vi "Send Open Front Panel.vi"(5 "Activate?":bool, 7 "Priority":T2=enum."Normal" caption="Message Priority (Normal)", 8 "error in (no error)":errorcluster, 9 "Front Panel Window:State":T1(ring), 10 "View Hierarchy Level":i32, 11 "Message Enqueuer in":refnum<class "Message Enqueuer.lvclass">) -> (0 "error out":errorcluster, 3 "Message Enqueuer out":refnum<class "Message Enqueuer.lvclass">)   [LabVIEW 2023, in "GUI Views.lvlib" / "Open Front Panel Msg.lvclass"]
doc: "Sends the <b>GUI Views.lvlib:Open Front Panel Msg.lvclass</b> message.\n\nThis message will call <b>Open Front Panel.vi</b> on the <b>GUI Views.lvlib:GUI View.lvclass</b> actor.\n\n<b>Open Front Panel.vi Description</b>\nOpens the Front Panel of a specified Actor Core VI of the the specified View class hierarchy. The method is active only if the GUI View is not contained. The Front Panel is specified by: \n\n<b> View Hierarchy Level</b> the level on the subclassing hierarchy of the GUI View actor, it is used to choose the Actor Core Front Panel among all the exisiting sublcasses of the GUI VIew Actor present in the View specified above"
uses:
  Open Front Panel Msg.lvclass
  Open Front Panel Msg.lvclass/Open Front Panel Msg.ctl
  <vilib>/ActorFramework/Message Enqueuer/Message Enqueuer.lvclass
  C:/Program Files/National Instruments/LabVIEW 2023/vi.lib/ActorFramework/Message/Message.lvclass
  C:/Projects/Shared Libraries/Event Actors/GUI Views/GUI View Messages/Open Front Panel Msg/Open Front Panel Msg.lvclass
  <vilib>/ActorFramework/Message Enqueuer/Message Priority.ctl
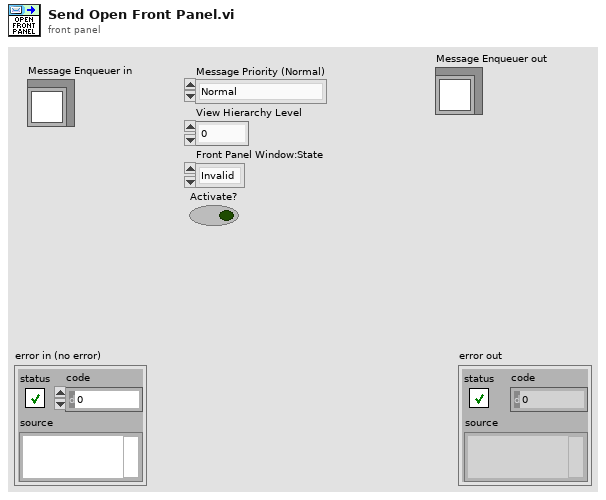
[diagram p1: front panel]
types:
  T1 = enum32{"Invalid", "Standard", "Closed", "Hidden", "Minimized", "Maximized"}
  T2 = typedef "Actor Framework.lvlib/Message Enqueuer.lvclass/Message Priority.ctl" = enum16{"Low", "Normal", "High"}
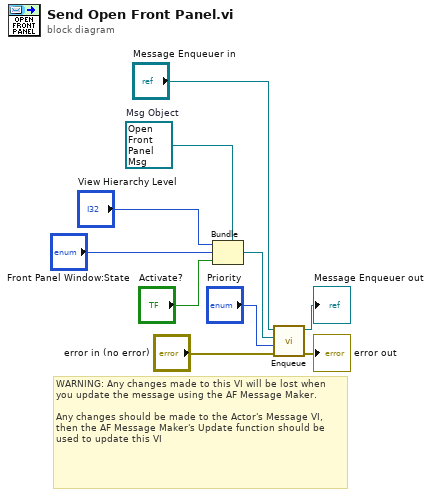
[diagram p0: block diagram]
diagram:
  w7 = refnum<class "Open Front Panel Msg.lvclass"> refnum  # Msg Object
  # "WARNING: Any changes made to this VI will be lost when you update the message using the AF Message Maker.\n\nAny changes should be made to the Actor's Message VI, then the AF Message Maker's Update function should be used to update this VI"
  n1 = Bundle(cluster=w7, "View Hierarchy Level", "Front Panel Window:State", "Activate?") -> (w2:refnum<class "Open Front Panel Msg.lvclass">)
  n2 = call <vilib>:"Enqueue.vi"("error in (no error)"="error in (no error)", "Message Priority (Normal)"="Priority", "Message"=w2, "Message Enqueuer in"="Message Enqueuer in") -> ("error out"=→"error out":errorcluster, "Message Enqueuer out"=→"Message Enqueuer out":refnum<class "Message Enqueuer.lvclass">)  [unwired: 6 in]
